vi "config_frec_amp.vi"(6 "Impedancia":string(combo), 8 "error in (no error)":errorcluster, 9 "Frec (Hz)":dbl, 10 "Amplitud (Vrms)":dbl) -> (0 "error out":errorcluster, 3 "DS360 out":refnum<class "DS360.lvclass">)   [LabVIEW 2019, in "DS360.lvclass"]
doc: "Configura el Generador con una frecuencia y amplitud conocida."
uses:
  DS360.lvclass
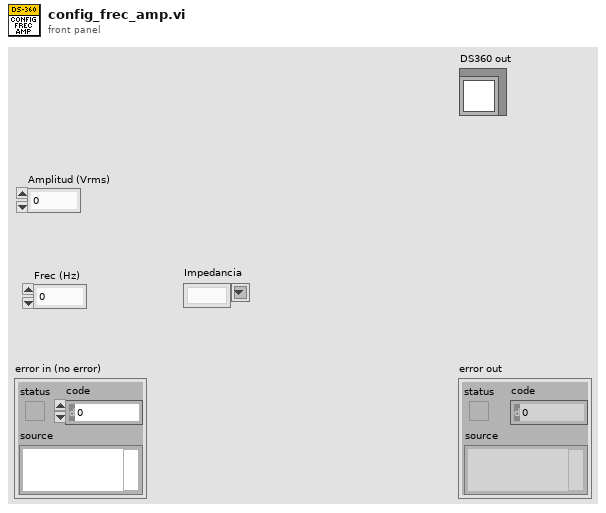
[diagram p1: front panel]
types:
  T1 = cluster{"error":bool, "code":i32, "source":string}
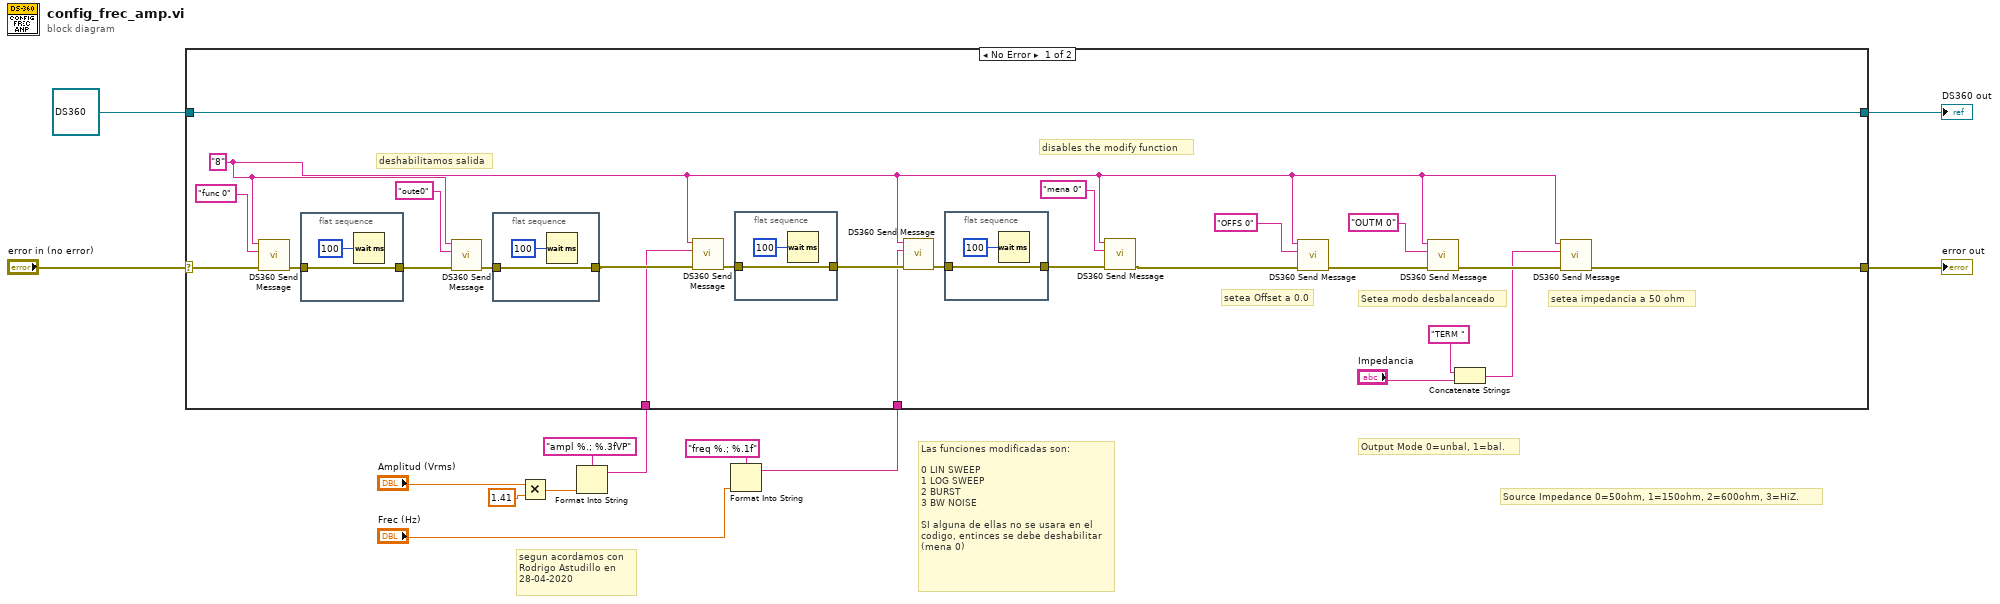
[diagram p0: block diagram]
diagram:
  # "Source Impedance 0=50ohm, 1=150ohm, 2=600ohm, 3=HiZ."
  # "Output Mode 0=unbal, 1=bal."
  # "Las funciones modificadas son:\n\n0 LIN SWEEP\n1 LOG SWEEP\n2 BURST\n3 BW NOISE\n\nSI alguna de ellas no se usara en el\ncodigo, entinces se debe deshabilitar\n(mena 0)"
  # "segun acordamos con\nRodrigo Astudillo en\n28-04-2020"
  n1 = Multiply(x="Amplitud (Vrms)", y=1.41) -> (x*y=w5:dbl)
  n2 = Format Into String(format string="ampl %.; %.3fVP" ("write buffer"), w5) -> (resulting string=w4:string)  [unwired: 2 in, 1 out]
  n3 = Format Into String(format string="freq %.; %.1f" ("write buffer"), "Frec (Hz)") -> (resulting string=w3:string)  [unwired: 2 in, 1 out]
  n4 = case shown="No Error" "error in (no error)" {
    selector: "error in (no error)" -> [w31 w47]
    tunnel: [w17 w47] -> w11
    tunnel: [w37 w46] -> w9
    tunnel: refnum<class "DS360.lvclass"> refnum ("DS360 in") -> [w37 w46]
    tunnel: w4 -> [w23 _]
    tunnel: w3 -> [w22 _]
    frame No Error {
      w16 = "8" ("write buffer")
      # "setea impedancia a 50 ohm"
      # "Setea modo desbalanceado"
      # "setea Offset a 0.0"
      # "disables the modify function"
      # "deshabilitamos salida"
      n5 = call <instrlib>:"DS360 Send Message.vi"("address string"=w16, "write buffer"="func 0", "error in"=w31) -> ("error out"=w34:T1)  [unwired: 3 in, 3 out]
      n6 = flat-sequence {
        tunnel: w34 -> [w45]
        tunnel: [w45] -> w33
        frame #0 {
          n7 = Wait (ms)(milliseconds to wait=u32 100) -> ()  [unwired: 1 out]
        }
      }
      n8 = call <instrlib>:"DS360 Send Message.vi"("address string"=w16, "write buffer"="oute0", "error in"=w33) -> ("error out"=w32:T1)  [unwired: 3 in, 3 out]
      n9 = flat-sequence {
        tunnel: w32 -> [w43]
        tunnel: [w43] -> w25
        frame #0 {
          n10 = Wait (ms)(milliseconds to wait=u32 100) -> ()  [unwired: 1 out]
        }
      }
      n11 = call <instrlib>:"DS360 Send Message.vi"("address string"=w16, "write buffer"=w23, "error in"=w25) -> ("error out"=w29:T1)  [unwired: 3 in, 3 out]
      n12 = flat-sequence {
        tunnel: w29 -> [w41]
        tunnel: [w41] -> w28
        frame #0 {
          n13 = Wait (ms)(milliseconds to wait=u32 100) -> ()  [unwired: 1 out]
        }
      }
      n14 = call <instrlib>:"DS360 Send Message.vi"("address string"=w16, "write buffer"=w22, "error in"=w28) -> ("error out"=w27:T1)  [unwired: 3 in, 3 out]
      n15 = flat-sequence {
        tunnel: w27 -> [w39]
        tunnel: [w39] -> w26
        frame #0 {
          n16 = Wait (ms)(milliseconds to wait=u32 100) -> ()  [unwired: 1 out]
        }
      }
      n17 = call <instrlib>:"DS360 Send Message.vi"("address string"=w16, "write buffer"="mena 0", "error in"=w26) -> ("error out"=w24:T1)  [unwired: 3 in, 3 out]
      n18 = call <instrlib>:"DS360 Send Message.vi"("address string"=w16, "write buffer"="OFFS 0", "error in"=w24) -> ("error out"=w20:T1)  [unwired: 3 in, 3 out]
      n19 = call <instrlib>:"DS360 Send Message.vi"("address string"=w16, "write buffer"="OUTM 0", "error in"=w20) -> ("error out"=w19:T1)  [unwired: 3 in, 3 out]
      n20 = Concatenate Strings("TERM " ("write buffer"), "Impedancia") -> (w13:string)
      n21 = call <instrlib>:"DS360 Send Message.vi"("address string"=w16, "write buffer"=w13, "error in"=w19) -> ("error out"=w17:T1)  [unwired: 3 in, 3 out]
    }
    frame Error {
    }
  }
  "error out" <- w11
  "DS360 out" <- w9
